vi "Write_GeneralAutoData.vi"(8 "error in (no error)":errorcluster, 10 "General Auto Data":T1, 11 "DriveAuto in":refnum<class "DriveAuto.lvclass">) -> (0 "error out":errorcluster, 3 "DriveAuto out":refnum<class "DriveAuto.lvclass">)   [LabVIEW 2017]
uses:
  DriveAuto.lvclass
  GeneralAutoData.ctl
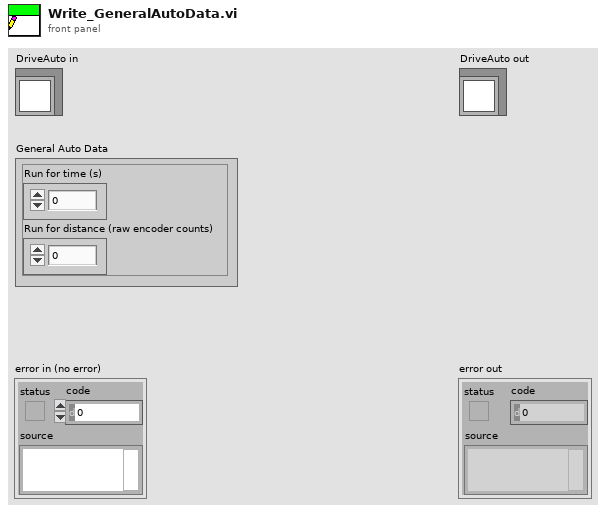
[diagram p1: front panel]
types:
  T1 = typedef "GeneralAutoData.ctl" = cluster{"Run for time (s)":dbl, "Run for distance (raw encoder counts)":dbl}
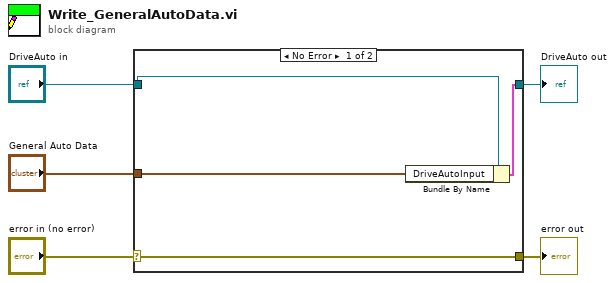
[diagram p0: block diagram]
diagram:
  n1 = case shown="No Error" "error in (no error)" {
    selector: "error in (no error)" -> [w9 w10]
    tunnel: [w9 w10] -> w4
    tunnel: [w7 w11] -> w2
    tunnel: "DriveAuto in" -> [w8 w11]
    tunnel: "General Auto Data" -> [w6 _]
    frame No Error {
      n2 = Bundle By Name(cluster=w8, "DriveAutoInput"=w6) -> (w7:cluster{})
    }
    frame Error {
    }
  }
  "error out" <- w4
  "DriveAuto out" <- w2
